vi "TriangularWave.vi"() -> ()   [LabVIEW 2014]
doc: "Shows how to set and get the piezo position."
panel:
  in  "amplitude":dbl=75.0
  in  "lMode":i32=2
  in  "Período":sgl=20.0
  in  "#Ciclos":i32=1
  in  "MG17Piezo":refnum<k7>(container)
  # "#1-Ondas continuas(Desconsiderar # de ciclos)\n#2-Ciclos determinados"
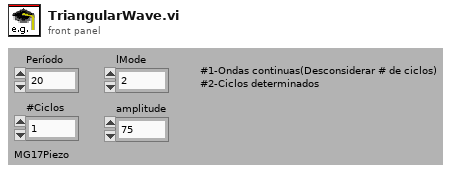
[diagram p1: front panel]
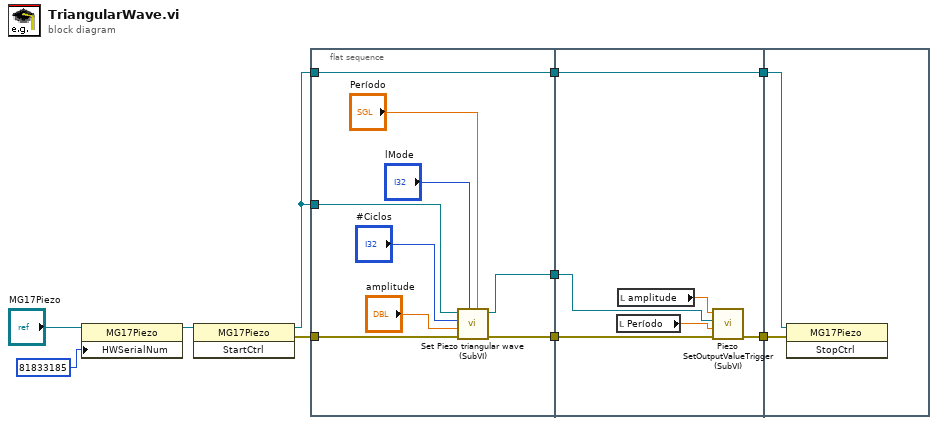
[diagram p0: block diagram]
diagram:
  n1 = property class="MG17Piezo"(reference="MG17Piezo", "HWSerialNum"=81833185) -> (reference out=w8:refnum<k7>)  [unwired: 1 in, 1 out]
  n2 = invoke class="MG17Piezo" method="StartCtrl"(reference=w8) -> (reference out=w2:refnum<k7>, error out=w7:errorcluster)  [unwired: 2 in, 1 out]
  n3 = flat-sequence {
    tunnel: w2 -> [w19]
    tunnel: w7 -> [w18]
    tunnel: [w17] -> w6
    tunnel: [w16] -> w5
    tunnel: w2 -> [w15]
    tunnel: [w15] -> w1
    tunnel: w6 -> [w24]
    tunnel: w5 -> [w25]
    tunnel: [w23] -> w4
    tunnel: [w22] -> w3
    tunnel: w1 -> [w22]
    tunnel: w4 -> [w27]
    tunnel: w3 -> [w26]
    frame #0 {
      n4 = call "Set Piezo triangular wave (SubVI).vi"("Período"="Período", "lMode"="lMode", "error in (no error)"=w18, "amplitude"="amplitude", "#Ciclos"="#Ciclos", "MG17Piezo in"=w19) -> ("error out"=w16:errorcluster, "MG17Piezo out"=w17:refnum<k7>)  [unwired: 4 in]
    }
    frame #1 {
      n5 = local read "Período"() -> (w20:sgl)
      n6 = local read "amplitude"() -> (w21:dbl)
      n7 = call "Piezo SetOutputValueTrigger (SubVI).vi"("error in (no error)"=w25, "Período"=w20, "MG17Piezo"=w24, "amplitude"=w21) -> ("error out"=w23:errorcluster)  [unwired: 7 in]
    }
    frame #2 {
      n8 = invoke class="MG17Piezo" method="StopCtrl"(reference=w26, error in=w27) -> ()  [unwired: 1 in, 3 out]
    }
  }
